vi "Configure System Reference Clock.vi"(8 "error in (no error)":errorcluster, 10 "Reference Clock Source (1: Auto)":i32(ring)=1 items=["Internal", "Auto"], 11 "Chassis VISA resource name":refnum<visa-resource-name>) -> (0 "error out":errorcluster, 3 "Chassis VISA resource name out":refnum<visa-resource-name>)   [LabVIEW 2018, in "Agilent U2722.lvlib"]
doc: "This VI selects the reference clock source.\n\n<B>Note: </B>\nThe VISA resouce name of this VI should be the 2781 chassis' VISA resource name."
uses:
  <instrlib>/Agilent U2722/Agilent U2722.lvlib
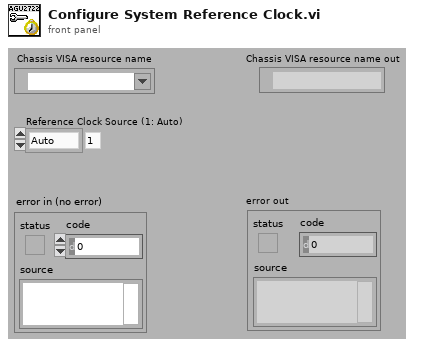
[diagram p1: front panel]
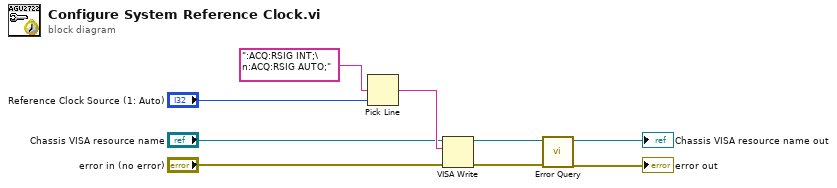
[diagram p0: block diagram]
diagram:
  n1 = Pick Line(multi-line string=":ACQ:RSIG INT;\n:ACQ:RSIG AUTO;", line index="Reference Clock Source (1: Auto)") -> (output string=w7:string)  [unwired: 1 out]
  n2 = VISA Write(VISA resource name="Chassis VISA resource name", write buffer=w7, error in (no error)="error in (no error)") -> (VISA resource name out=w4:refnum<visa-resource-name>, error out=w3:errorcluster)  [unwired: 1 out]
  n3 = call <instrlib>:"Error Query.vi"("error in (no error)"=w3, "VISA resource name"=w4) -> ("error out"=→"error out":errorcluster, "VISA resource name out"=→"Chassis VISA resource name out":refnum<visa-resource-name>)  [unwired: 6 in, 2 out]
